vi "FailTest.vi"(10 "Fail Test":bool, 11 "TestCaseMock in":refnum<class "TestCaseMock.lvclass">) -> (3 "TestCaseMock out":refnum<class "TestCaseMock.lvclass">)   [LabVIEW 2019, in "TestResultTestSupport.lvlib" / "TestCaseMock.lvclass"]
uses:
  TestCaseMock.lvclass
  TestCaseMock.lvclass/TestCaseMock.ctl
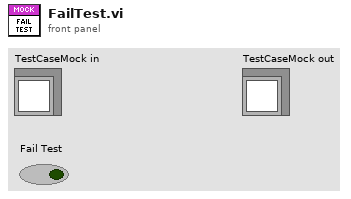
[diagram p1: front panel]
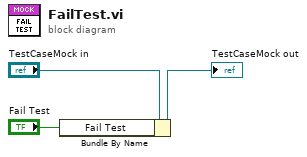
[diagram p0: block diagram]
diagram:
  n1 = Bundle By Name(cluster="TestCaseMock in", "Fail Test"="Fail Test") -> (→"TestCaseMock out":refnum<class "TestCaseMock.lvclass">)
